vi "Get Status.vi"() -> (0 "FPGA Timekeeper locked":bool, 1 "offset from time reference":i32)   [LabVIEW 2020, in "FPGA Timekeeper.lvlib"]
doc: "Provides the status of the current state of the FPGA Timekeeper."
uses:
  FPGA Timekeeper.lvlib
  private/timekeeper locked (g).vi
  private/offset from timeref (g).vi
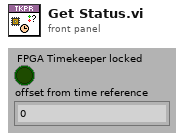
[diagram p1: front panel]
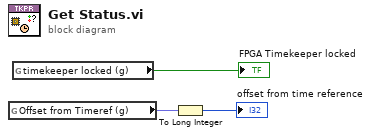
[diagram p0: block diagram]
diagram:
  n1 = global read "offset from timeref (g).vi" "Offset from Timeref (g)"() -> (w3:fxp<+/-,21,21>)
  n2 = global read "timekeeper locked (g).vi" "timekeeper locked (g)"() -> (→"FPGA Timekeeper locked":bool)
  n3 = To Long Integer(number=w3) -> (32bit integer=→"offset from time reference":i32)
